vi "unpack1byte.vi"(1 "ID":u8[](array[numeric])=[16, 32] format="%x") -> (0 "number":u32)   [LabVIEW 2020]
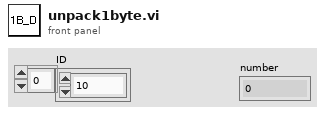
[diagram p1: front panel]
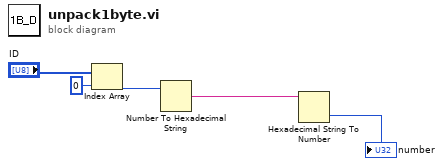
[diagram p0: block diagram]
diagram:
  n1 = Index Array(array="ID", index=0) -> (element=w4:u8)
  n2 = Number To Hexadecimal String(2:w4) -> (0:w1:string)  [unwired: 1 in]
  n3 = Hexadecimal String To Number(string=w1) -> (number=→"number":u32)  [unwired: 2 in, 1 out]
